vi "Wait For OPC.vi"(8 "error in (no error)":errorcluster {"code" format="%.0x"}, 10 "Timeout (10000 ms)":i32=10000, 11 "VISA resource name":refnum<visa-resource-name>) -> (0 "error out":errorcluster {"code" format="%.0x"}, 2 "Complete":bool, 3 "VISA resource name out":refnum<visa-resource-name>)   [LabVIEW 2019, in "Pendulum CNT90.lvlib"]
doc: "This VI waits for end of measurement."
uses:
  Pendulum CNT90.lvlib
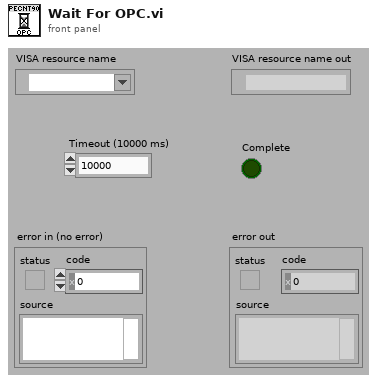
[diagram p1: front panel]
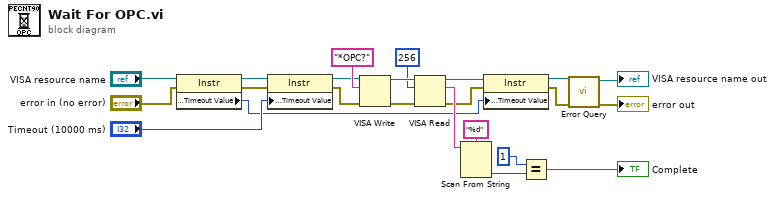
[diagram p0: block diagram]
diagram:
  n1 = property class="Instr"(reference="VISA resource name", error in="error in (no error)") -> (reference out=w10:refnum<visa-resource-name>, error out=w9:errorcluster, "General Settings:Timeout Value"=w1:u32)
  n2 = property class="Instr"(reference=w10, error in=w9, "General Settings:Timeout Value"="Timeout (10000 ms)") -> (reference out=w7:refnum<visa-resource-name>, error out=w6:errorcluster)
  n3 = VISA Write(VISA resource name=w7, write buffer="*OPC?", error in (no error)=w6) -> (VISA resource name out=w19:refnum<visa-resource-name>, error out=w18:errorcluster)  [unwired: 1 out]
  n4 = VISA Read(VISA resource name=w19, byte count=u32 256, error in (no error)=w18) -> (VISA resource name out=w5:refnum<visa-resource-name>, read buffer=w16:string, error out=w4:errorcluster)  [unwired: 1 out]
  n5 = Scan From String(format string="%d", input string=w16) -> (output 1=w14:i32)  [unwired: 3 in, 3 out]
  n6 = property class="Instr"(reference=w5, error in=w4, "General Settings:Timeout Value"=w1) -> (reference out=w2:refnum<visa-resource-name>, error out=w3:errorcluster)
  n7 = Equal?(x=1, y=w14) -> (x = y?=→"Complete":bool)
  n8 = call "Error Query.vi"("error in (no error)"=w3, "VISA resource name"=w2) -> ("error out"=→"error out":errorcluster, "VISA resource name out"=→"VISA resource name out":refnum<visa-resource-name>)  [unwired: 6 in, 2 out]
